vi "Construct.vi"(8 "error in (no error)":errorcluster, 11 "Database Connection":T1={"Database Driver"="PostgreSQL Unicode", "Server"="127.0.0.1", "Port"=5432, "Database"="postgres", "User ID"="postgres", "Password"="postgres"}) -> (0 "error out":errorcluster, 3 "SLL Database out":refnum<class "SLL Database.lvclass">)   [LabVIEW 2014, in "SLL Database.lvclass"]
doc: "Initializes a database connection and constructs the database object"
uses:
  SLL Database.lvclass
  SLL Database.lvclass/SLL Database.ctl
  <vilib>/addons/database/Connection.llb/DB Tools Open Connec (String).vi
  <vilib>/addons/database/NI_Database_API.lvlib
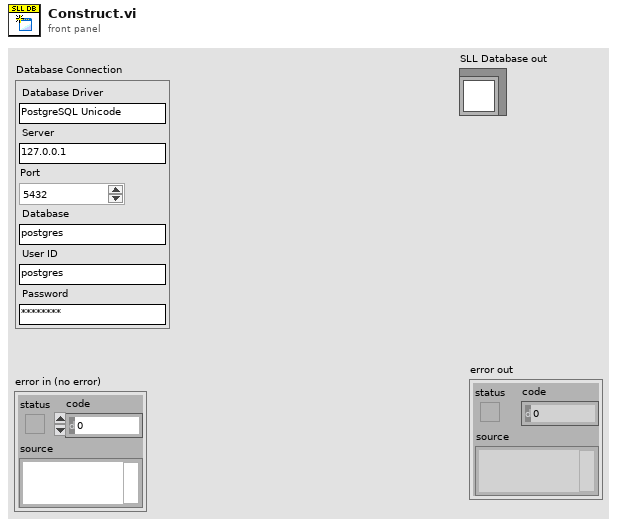
[diagram p1: front panel]
types:
  T1 = cluster{"Database Driver":string, "Server":string, "Port":i32, "Database":string, "User ID":string, "Password":string}
  T2 = typedef "NI_Database_API.lvlib/Conn ObjectReference.ctl" = refnum<k1>
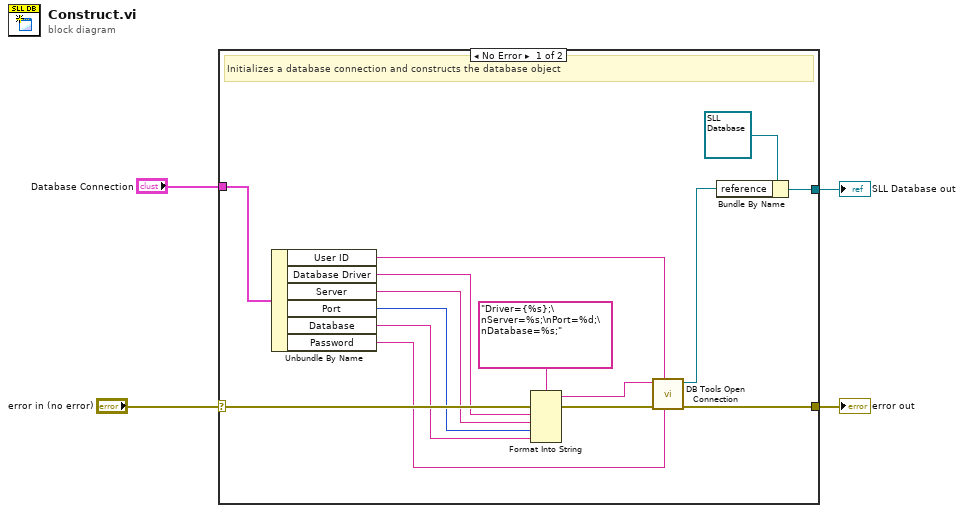
[diagram p0: block diagram]
diagram:
  n1 = case shown="No Error" "error in (no error)" {
    selector: "error in (no error)" -> [w19 w20]
    tunnel: [w18 w20] -> w3
    tunnel: [w15 _] -> w2
    tunnel: "Database Connection" -> [w12 _]
    frame No Error {
      # "Initializes a database connection and constructs the database object"
      n2 = Unbundle By Name(w12) -> ("User ID"=w10:string, "Database Driver"=w9:string, "Server"=w8:string, "Port"=w7:i32, "Database"=w6:string, "Password"=w5:string)
      n3 = Format Into String(format string="Driver={%s};\nServer=%s;\nPort=%d;\nDatabase=%s;", error in=w19, w9, w8, w7, w6) -> (resulting string=w11:string, error out=w14:errorcluster)  [unwired: 1 in]
      n4 = call-poly <vilib>:"DB Tools Open Connection.vi"("password"=w5, "userID"=w10, "error in (no error)"=w14, "connection information"=w11) -> ("error out"=w18:errorcluster, "connection reference"=w16:T2)  [unwired: 4 in]
      n5 = Bundle By Name(cluster=refnum<class "SLL Database.lvclass"> refnum ("SLL Database out"), "reference"=w16) -> (w15:refnum<class "SLL Database.lvclass">)
    }
    frame Error {
    }
  }
  "error out" <- w3
  "SLL Database out" <- w2
